vi "(SubVI) Marko-Sigga WLC fitting and deal with center and force shift.vi"(3 "Force (pN)":dbl[](array[numeric]), 4 "Extension (nm)":dbl[](array[numeric]), 6 "initial parameters for marko":dbl[](array[numeric])=[40.0, 1800.0, 0.001, 0.001]) -> (0 "best nonlinear fit for Force (pN)":dbl[](array[numeric]), 1 "r^2":dbl, 2 "best fit parameters\n(Lp,Lc,dL,dF)":dbl[](array[numeric]))   [LabVIEW 2014]
uses:
  <vilib>/gmath/NumericalOptimization/Nonlinear Curve Fit LM formula string.vi
  <vilib>/gmath/NI_Gmath.lvlib
panel:
  out "error out":errorcluster
  out "residue":dbl
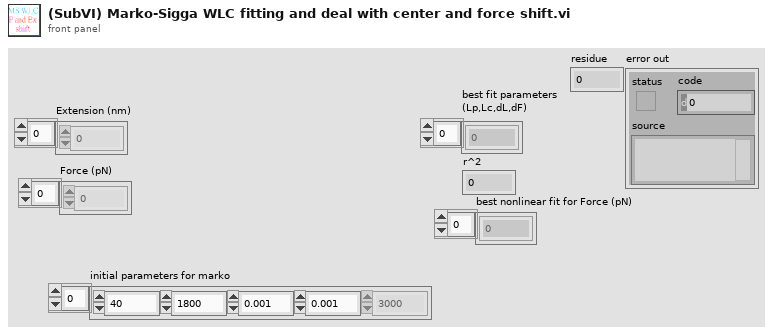
[diagram p1: front panel]
types:
  T1 = cluster{"model":string, "Parameters":string[], "x":string}
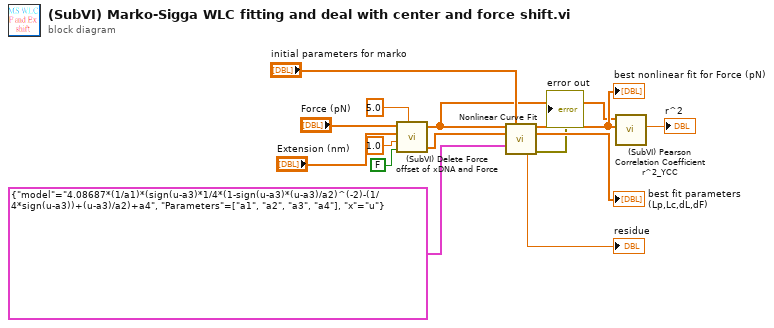
[diagram p0: block diagram]
diagram:
  n1 = call "(SubVI) Delete Force offset of xDNA and Force.vi"("Force"="Force (pN)", "Upper Force (pN)"=5.0, "xDNA"="Extension (nm)", "force constant"=1.0, "Set lower foce offset?"=FALSE) -> ("cut-full Force"=w3:dbl[], "cut-full xDNA"=w2:dbl[])  [unwired: 2 in]
  n2 = call-poly <vilib>:"Nonlinear Curve Fit.vi"("Y"=w3, "initial parameters"="initial parameters for marko", "X"=w2, "model description"=T1 {"model"="4.08687*(1/a1)*(sign(u-a3)*1/4*(1-sign(u-a3)*(u-a3)/a2)^(-2)-(1/4*sign(u-a3))+(u-a3)/a2)+a4", "Parameters"=["a1", "a2", "a3", "a4"], "x"="u"}) -> ("best nonlinear fit"=w10:dbl[], "best fit parameters"=→"best fit parameters\n(Lp,Lc,dL,dF)":dbl[], "residue"=→"residue":dbl, "error out"=→"error out":errorcluster)  [unwired: 3 in, 5 out]
  "best nonlinear fit for Force (pN)" <- w10
  n3 = call "(SubVI) Pearson Correlation Coefficient r^2_YCC.vi"("best fit Data"=w10, "Data"=w3) -> ("r^2"=→"r^2":dbl)  [unwired: 4 in, 1 out]
